vi "get time stamp.vi"(8 "error in (no error)":errorcluster, 11 "PCO_Camera in":refnum<class "PCO_Camera.lvclass">) -> (0 "error out":errorcluster, 3 "PCO_Camera out":refnum<class "PCO_Camera.lvclass">)   [LabVIEW 2020, in "PCO_Camera.lvclass"]
uses:
  PCO_Camera.lvclass
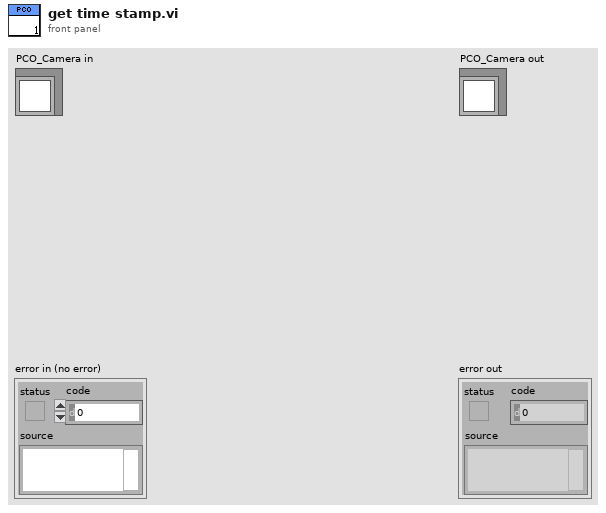
[diagram p1: front panel]
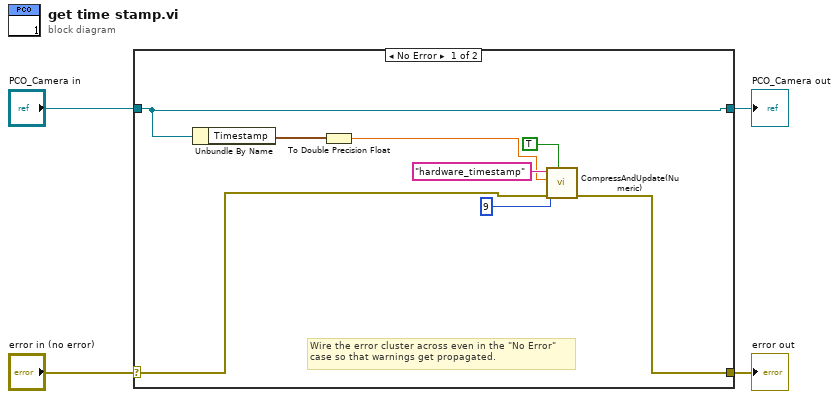
[diagram p0: block diagram]
diagram:
  n1 = case shown="No Error" "error in (no error)" {
    selector: "error in (no error)" -> [w7 w14]
    tunnel: [w6 w14] -> w3
    tunnel: [w5 w13] -> w1
    tunnel: "PCO_Camera in" -> [w5 w13]
    frame No Error {
      # "Wire the error cluster across even in the \"No Error\"\ncase so that warnings get propagated."
      n2 = Unbundle By Name(w5) -> ("Timestamp"=w12:timestamp)
      n3 = To Double Precision Float(number=w12) -> (double precision float=w8:dbl)
      n4 = call "CompressAndUpdate(Numeric).vi"("force CVT update (false)"=TRUE, "error in"=w7, "precision (6)"=i16 9, "Numeric"=w8, "command or variable name"="hardware_timestamp") -> ("error out"=w6:errorcluster)  [unwired: 6 in]
    }
    frame Error {
    }
  }
  "error out" <- w3
  "PCO_Camera out" <- w1
